vi "s2.vi"() -> ()   [LabVIEW 2017]
panel:
  in  "Period, s":dbl(slide) scale=0.01..10.0
  in  "stop":bool
  out "Waveform Chart":cluster{"number: 0 to 1":dbl, dbl}(graph)
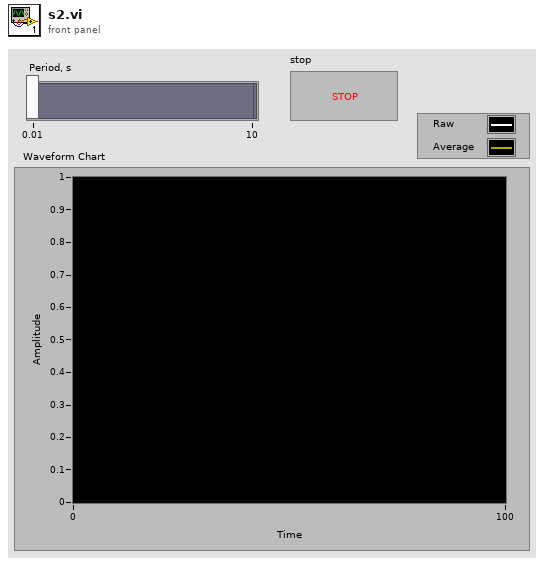
[diagram p1: front panel]
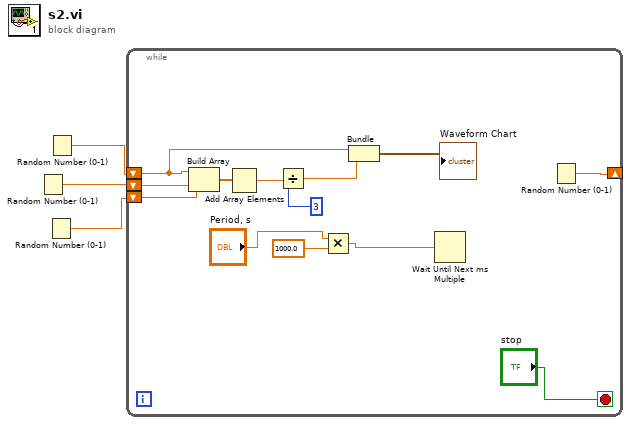
[diagram p0: block diagram]
diagram:
  n1 = Random Number (0-1)() -> (number: 0 to 1=w2:dbl)
  n2 = Random Number (0-1)() -> (number: 0 to 1=w3:dbl)
  n3 = Random Number (0-1)() -> (number: 0 to 1=w1:dbl)
  n4 = while {
    shift-right: [w12] -> _
    shift-left: w3 -> [w11]
    shift-left: w2 -> [w10]
    shift-left: w1 -> [w8]
    stop <- "stop" stop-if-true
    n5 = Build Array(w8, w10, w11) -> (w9:dbl[])
    n6 = Add Array Elements(numeric array=w9) -> (sum=w4:dbl)
    n7 = Divide(x=w4, y=3) -> (x/y=w7:dbl)
    n8 = Multiply(x="Period, s", y=1000.0) -> (x*y=w13:dbl)
    n9 = Bundle("number: 0 to 1"=w8, w7) -> (→"Waveform Chart":cluster{"number: 0 to 1":dbl, dbl})  [unwired: 1 in]
    n10 = Wait Until Next ms Multiple(millisecond multiple=w13) -> ()  [unwired: 1 out]
    n11 = Random Number (0-1)() -> (number: 0 to 1=w12:dbl)
  }
